vi "Flatten to YAML.vi"(8 "error in (no error)":errorcluster, 11 "YAML Parser in":refnum<class "YAML Parser.lvclass">) -> (0 "error out":errorcluster, 2 "YAML String":string, 3 "YAML Parser out":refnum<class "YAML Parser.lvclass">)   [LabVIEW 2015, in "YAML Parser.lvclass"]
uses:
  YAML Parser.lvclass
  YAML Parser.lvclass/YAML Parser.ctl
  YAML Parser.lvlib
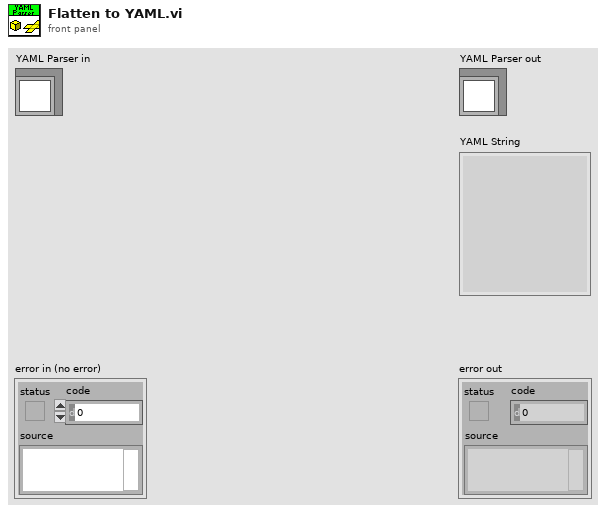
[diagram p1: front panel]
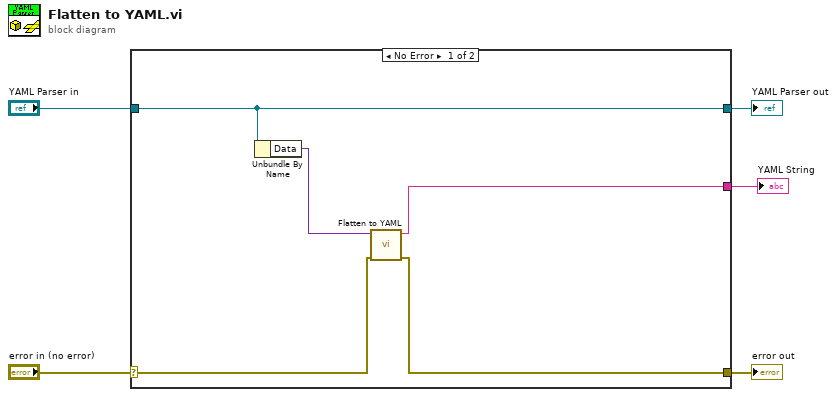
[diagram p0: block diagram]
diagram:
  n1 = case shown="No Error" "error in (no error)" {
    selector: "error in (no error)" -> [w10 w12]
    tunnel: [w9 w12] -> w4
    tunnel: [w8 w11] -> w2
    tunnel: "YAML Parser in" -> [w8 w11]
    tunnel: [w6 _] -> w1
    frame No Error {
      n2 = Unbundle By Name(w8) -> ("Data"=w7:variant)
      n3 = call "Flatten to YAML.vi"("error in (no error)"=w10, "Anything"=w7) -> ("error out"=w9:errorcluster, "YAML String"=w6:string)  [unwired: 8 in]
    }
    frame Error {
    }
  }
  "error out" <- w4
  "YAML Parser out" <- w2
  "YAML String" <- w1
